vi "Show Table.vi"(0 "Table":refnum<vi>, 7 "Data":T1, 11 "max rows":i32) -> (8 "items":i32[](array[numeric]))   [LabVIEW 2020, in "KPropertyTable.xctl"]
uses:
  KPropertyTable.xctl
  Data.vi
  RowData.ctl
  DataType.ctl
  Array Manipulation VIs/Array-Dimensions (2D string).vi
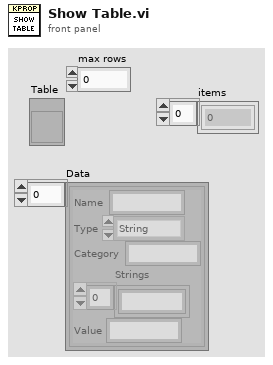
[diagram p1: front panel]
types:
  T1 = typedef "KPropertyTable.xctl/Data.vi" = T2[]
  T2 = typedef "KPropertyTable.xctl/RowData.ctl" = cluster{"Name":string, "Type":T3, "Category":string, "Strings":string[], "Value":string}
  T3 = typedef "KPropertyTable.xctl/DataType.ctl" = enum16{"String", "Enum", "Int", "Double", "Boolean", "Ring", "Formula"}
  T4 = cluster{u32, "Active Cell:Cell Font:Bold":bool}[]
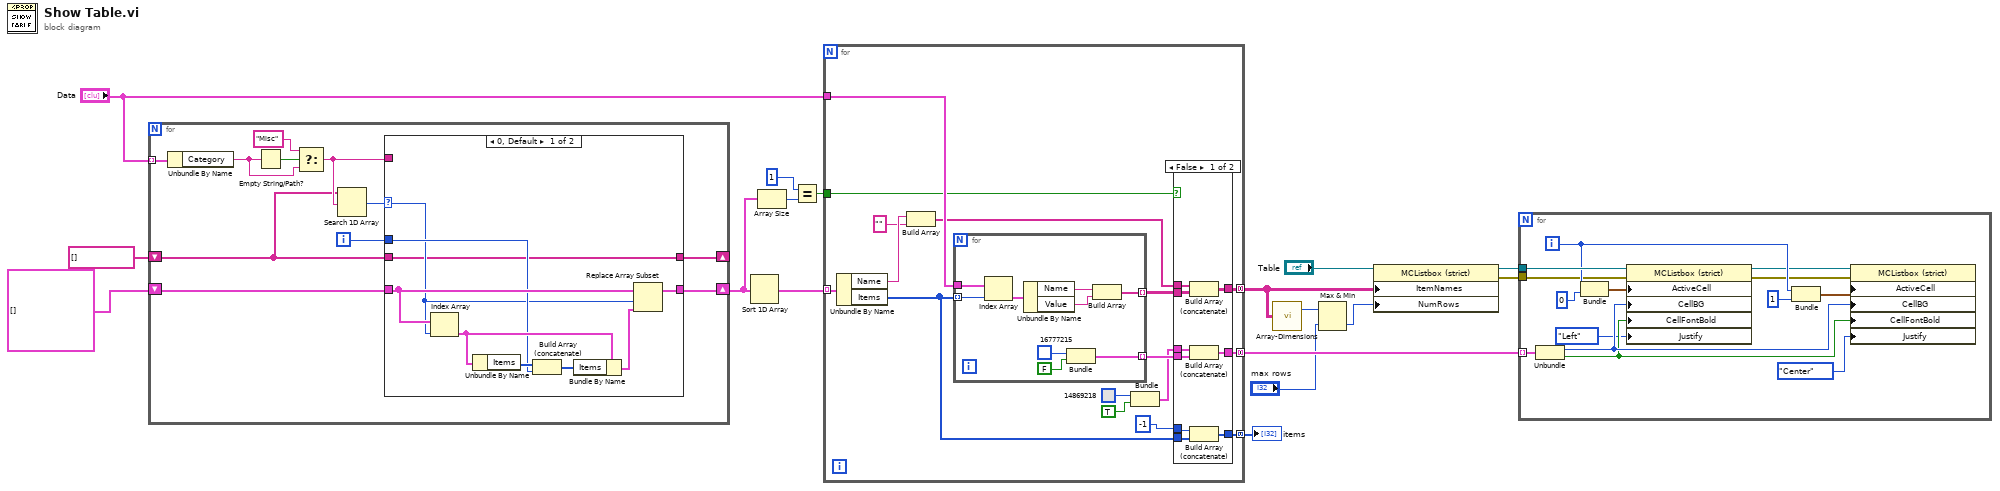
[diagram p0: block diagram]
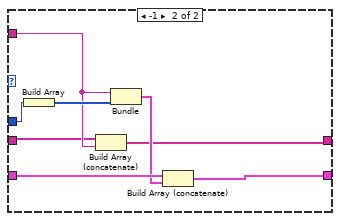
[diagram p3: hidden frame]
diagram:
  n1 = for {
    tunnel: "Data" -> [w28] mode=indexing
    shift-right: [w19] -> _
    shift-left: string[] [] -> [w18]
    shift-right: [w20] -> w7
    shift-left: cluster{"Name":string, "Items":i32[]}[] [] -> [w21]
    i -> [w22]
    n2 = Unbundle By Name(w28) -> ("Category"=w26:string)
    n3 = Empty String/Path?(string/path=w26) -> (empty?=w27:bool)
    n4 = Select(t="Misc", s=w27, f=w26) -> (s? t:f=w24:string)
    n5 = Search 1D Array(1D array=w18, element=w24) -> (index of element=w23:i32)  [unwired: 1 in]
    n6 = case shown="0, Default" w23 {
      selector: w23 -> [w30 _]
      tunnel: w24 -> [_ w40]
      tunnel: w22 -> [w31 w45]
      tunnel: w21 -> [w35 w43]
      tunnel: [w36 w41] -> w20
      tunnel: [w29 w38] -> w19
      tunnel: w18 -> [w29 w39]
      frame 0, Default {
        n7 = Index Array(array=w35, index=w30) -> (element=w34:cluster{"Name":string, "Items":i32[]})
        n8 = Unbundle By Name(w34) -> ("Items"=w37:i32[])
        n9 = Build Array (concatenate)(w37, w31) -> (w33:i32[])
        n10 = Bundle By Name(cluster=w34, "Items"=w33) -> (w32:cluster{"Name":string, "Items":i32[]})
        n11 = Replace Array Subset(array=w35, new element=w32, index=w30) -> (w36:cluster{"Name":string, "Items":i32[]}[])
      }
      frame -1 {
        n12 = Build Array(w45) -> (w44:i32[])
        n13 = Build Array (concatenate)(w39, w40) -> (w38:string[])
        n14 = Bundle("Category"=w40, w44) -> (w42:cluster{"Category":string, i32[]})  [unwired: 1 in]
        n15 = Build Array (concatenate)(w43, w42) -> (w41:cluster{"Category":string, "Items":i32[]}[])
      }
    }
  }
  n16 = Sort 1D Array(array=w7) -> (sorted array=w15:cluster{"Name":string, "Items":i32[]}[])
  n17 = Array Size(array=w7) -> (size(s)=w6:i32)
  n18 = Equal?(x=1, y=w6) -> (x = y?=w4:bool)
  n19 = for {
    tunnel: w15 -> [w61] mode=indexing
    tunnel: "Data" -> [w59]
    tunnel: [w56] -> w8 mode=concatenating
    tunnel: [w53] -> w12 mode=concatenating
    tunnel: [w46] -> w10 mode=concatenating
    tunnel: w4 -> [w49]
    n20 = Unbundle By Name(w61) -> ("Name"=w60:string, "Items"=w48:i32[])
    n21 = Build Array(w60, "") -> (w57:string[])
    n22 = for {
      tunnel: w48 -> [w82] mode=indexing
      tunnel: w59 -> [w81]
      tunnel: [w77] -> w58 mode=indexing
      tunnel: [w74] -> w55 mode=indexing
      n23 = Index Array(array=w81, index=w82) -> (element=w80:T2)
      n24 = Unbundle By Name(w80) -> ("Name"=w79:string, "Value"=w78:string)
      n25 = Bundle(u32 16777215, "Active Cell:Cell Font:Bold"=FALSE) -> (w74:cluster{u32, "Active Cell:Cell Font:Bold":bool})  [unwired: 1 in]
      n26 = Build Array(w79, w78) -> (w77:string[])
    }
    n27 = Bundle(u32 14869218, "Active Cell:Cell Font:Bold"=TRUE) -> (w54:cluster{u32, "Active Cell:Cell Font:Bold":bool})  [unwired: 1 in]
    n28 = case shown="False" w49 {
      tunnel: w58 -> [w70 w73]
      tunnel: w57 -> [w69 _]
      tunnel: [w68 w73] -> w56
      tunnel: w55 -> [w67 w72]
      tunnel: w54 -> [w66 _]
      tunnel: [w65 w72] -> w53
      tunnel: w48 -> [w64 w71]
      tunnel: -1 -> [w63 _]
      tunnel: [w62 w71] -> w46
      frame False {
        n29 = Build Array (concatenate)(w69, w70) -> (w68:string[][])
        n30 = Build Array (concatenate)(w66, w67) -> (w65:T4)
        n31 = Build Array (concatenate)(w63, w64) -> (w62:i32[])
      }
      frame True {
      }
    }
  }
  "items" <- w10
  n32 = call-poly "Array-Dimensions.vi"("2D Array"=w8) -> ("# rows"=w2:i32)  [unwired: 13 in, 1 out]
  n33 = Max & Min(x=w2, y="max rows") -> (min(x,y)=w1:i32)  [unwired: 1 out]
  n34 = property class="MCListbox (strict)"(reference="Table", "ItemNames"=w8, "NumRows"=w1) -> (reference out=w13:refnum<vi>, error out=w11:errorcluster)  [unwired: 1 in]
  n35 = for {
    tunnel: w13 -> [w94]
    tunnel: w12 -> [w93] mode=indexing
    tunnel: w11 -> [w90]
    i -> [w92]
    n36 = Unbundle(w93) -> (w86:u32, "Active Cell:Cell Font:Bold"=w85:bool)
    n37 = Bundle(w92, 0) -> (w96:cluster{i32, i32})  [unwired: 1 in]
    n38 = property class="MCListbox (strict)"(reference=w94, error in=w90, "ActiveCell"=w96, "CellBG"=w86, "CellFontBold"=w85, "Justify"=enum16{"Left", "Center", "Right"}."Left" ("Active Cell:Cell Justification")) -> (reference out=w91:refnum<vi>, error out=w89:errorcluster)
    n39 = Bundle(w92, 1) -> (w87:cluster{i32, i32})  [unwired: 1 in]
    n40 = property class="MCListbox (strict)"(reference=w91, error in=w89, "ActiveCell"=w87, "CellBG"=w86, "CellFontBold"=w85, "Justify"=enum16{"Left", "Center", "Right"}."Center" ("Active Cell:Cell Justification")) -> ()  [unwired: 2 out]
  }
